vi "FTW-Message-Construct.vi"(5 "RouterID":i64 format="%016x", 7 "Backtrace":string, 9 "Incoming Message":string, 11 "error in":errorcluster) -> (4 "FTW Incoming Message":refnum<class "FTW-Message.lvclass">, 15 "error out":errorcluster)   [LabVIEW 2013, in "FTW-Message.lvclass"]
uses:
  FTW-Message.lvclass
  FTW-Message.lvclass/FTW-Message.ctl
panel:
  # "Inputs"
  # "Outputs"
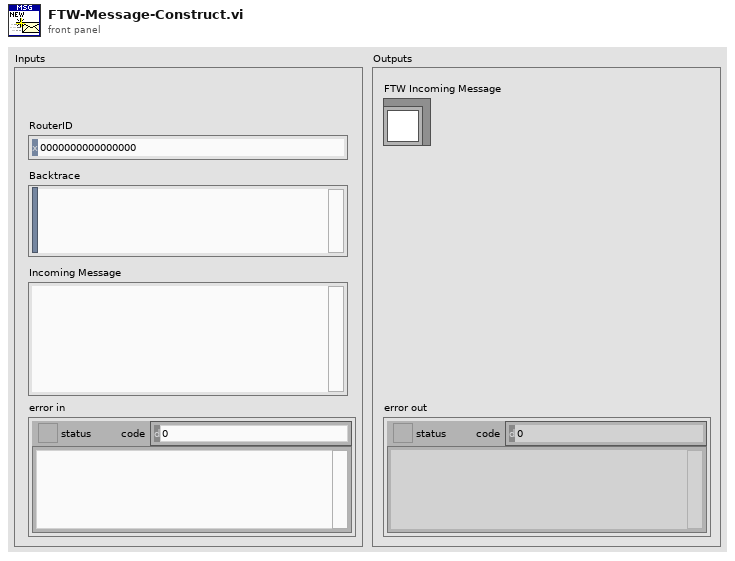
[diagram p1: front panel]
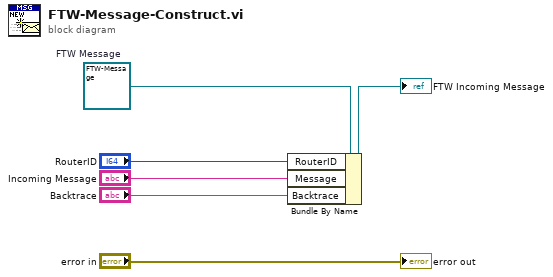
[diagram p0: block diagram]
diagram:
  w6 = refnum<class "FTW-Message.lvclass"> refnum  # FTW Message
  n1 = Bundle By Name(cluster=w6, "RouterID"="RouterID", "Message"="Incoming Message", "Backtrace"="Backtrace") -> (→"FTW Incoming Message":refnum<class "FTW-Message.lvclass">)
  "error out" <- "error in"
